vi "BusUI.vi"() -> ()   [LabVIEW 2014, in "Bus.lvclass"]
doc: "UI that will be called when the node is selected."
uses:
  Bus.lvclass
  <vilib>/NI/Configuration Framework/Node/NodeRef.ctl
  <vilib>/NI/Configuration Framework/Node/NISE_CEF_Node.lvclass
  <vilib>/NI/AMC/Message Queue.ctl
  <vilib>/NI/AMC/Message.ctl
  <vilib>/NI/Tools/Keyed Array/KeyedArray.ctl
  <vilib>/NI/Configuration Framework/Node/UserEventRef.ctl
  <vilib>/NI/Configuration Framework/Controls/EventCluster.ctl
  RIO Target/RIO Target.lvclass
  <vilib>/NI/Configuration Framework/Node/NISE_CEF_Node.lvclass/NISE_CEF_Node.ctl
  Bus.lvclass/Bus.ctl
  Bus Configuration/SPI Configuration.ctl
  Bus Configuration/Bus Configuration.lvclass/Bus Configuration.ctl
  <vilib>/NI/AMC/Create Single Message.vi
  <vilib>/NI/AMC/Update Message Routing Info.vi
  <vilib>/NI/AMC/Send Message.vi
  <vilib>/NI/AMC/AMC.lvlib
  <vilib>/NI/Configuration Framework/serializable configuration/NISE_CEF_serializable configuration.lvclass
  Bus Configuration/Bus Configuration.lvclass
  <vilib>/NI/Tools/Keyed Array/Tools_KeyedArray.lvlib
  <vilib>/NI/Configuration Framework/NISE_CEF_TreeControl.lvlib
panel:
  in  "Comments":string
  in  "SPI Engine":path
  in  "Driver Logic Unit":path
  in  "MOSI":string(combo)
  in  "MISO":string(combo)
  in  "SCLK":string(combo)
  in  "Alias":string
  in  "Replace Default SPI Engine?":bool
  in  "Replace Default DLU?":bool
  in  "user event":T1
  in  "main queue":T2
  in  "node ref":T3
  # "Settings"
  # "Alias"
  # "Comments"
  # "SPI Configuration"
  # "SCLK"
  # "SPI Engine"
  # "Driver Logic Unit"
  # "MOSI"
  # "MISO"
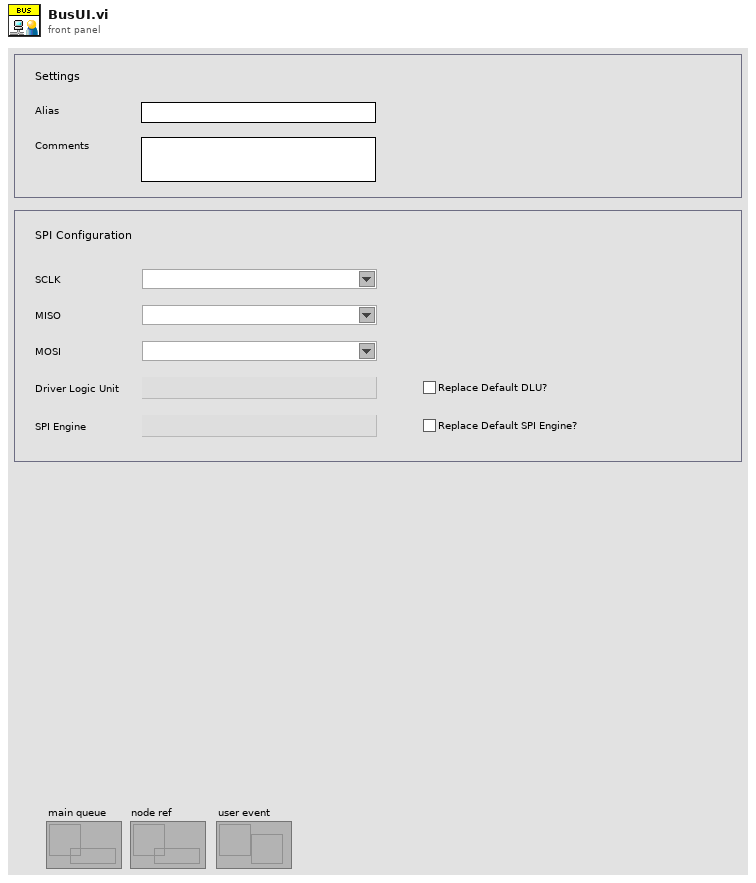
[diagram p1: front panel]
types:
  T1 = typedef "NISE_CEF_Node.lvclass/UserEventRef.ctl" = refnum<user-event>
  T2 = typedef "AMC.lvlib/Message Queue.ctl" = refnum<queue>
  T3 = typedef "NISE_CEF_Node.lvclass/NodeRef.ctl" = refnum<data-value>
  T4 = typedef "Bus.lvclass/UI Configuration.ctl" = cluster{"SPI Engine":path, "Driver Logic Unit":path, "alias":string, "SPI Configuration":T5, "Replace Default DLU?":bool, "Replace Default SPI Engine?":bool}
  T5 = typedef "Bus Configuration.lvclass/SPI Configuration.ctl" = cluster{"SCLK":string, "MOSI":string, "MISO":string}
  T6 = enum8{"Enabled", "Disabled", "Disabled and Grayed Out"}
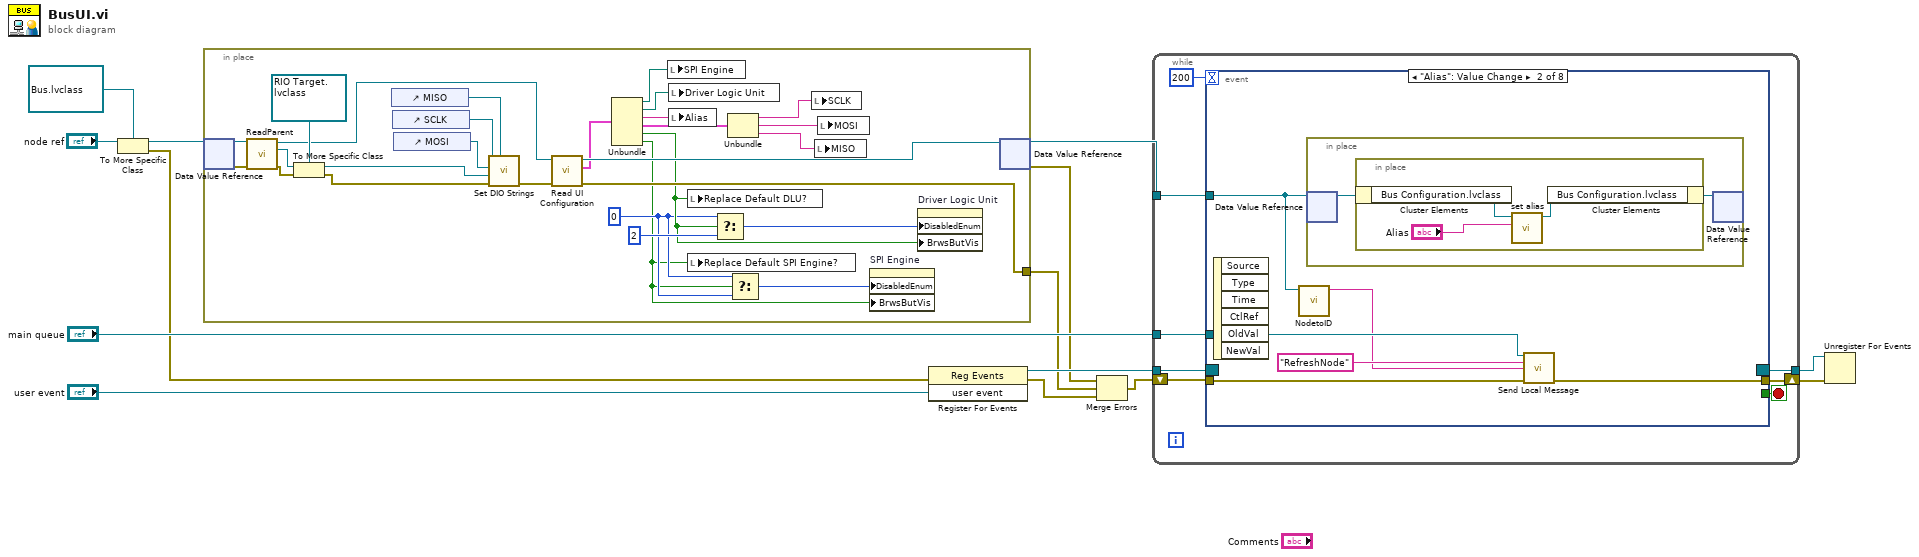
[diagram p0: block diagram]
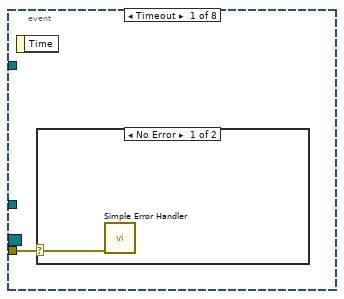
[diagram p2: hidden frame]
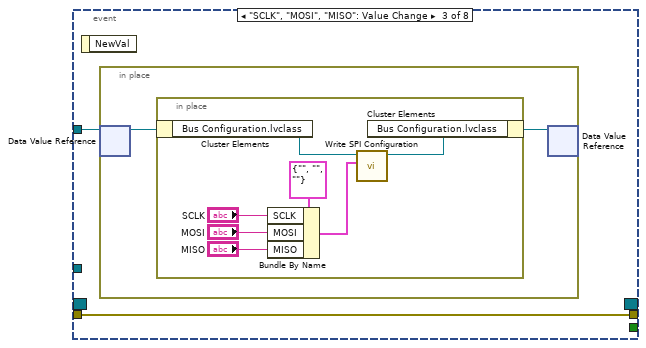
[diagram p4: hidden frame]
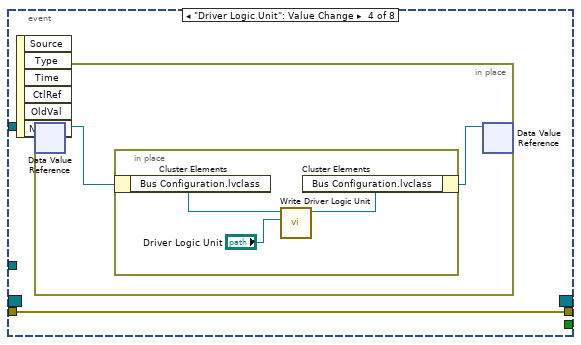
[diagram p5: hidden frame]
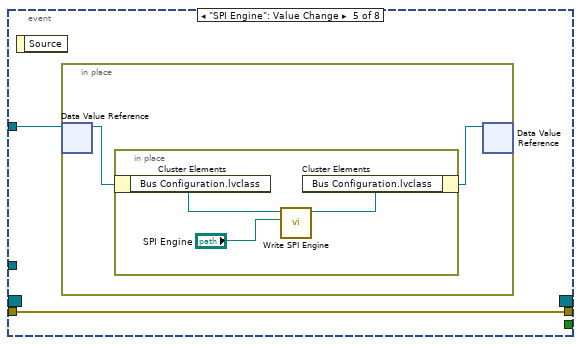
[diagram p6: hidden frame]
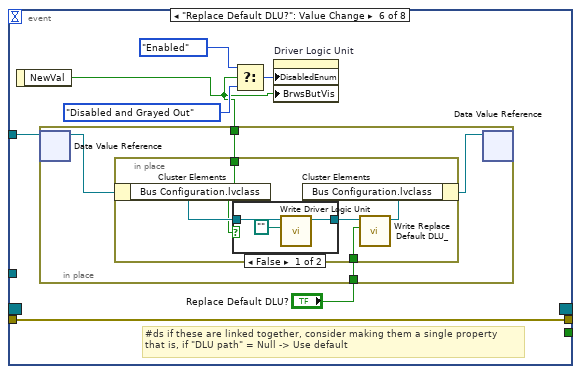
[diagram p7: hidden frame]
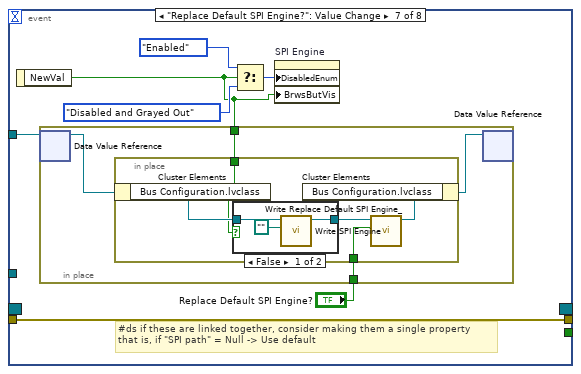
[diagram p9: hidden frame]
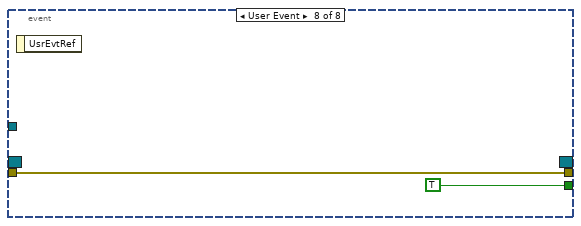
[diagram p11: hidden frame]
diagram:
  n1 = To More Specific Class(target class=refnum<data-value> refnum ("data value reference"), reference="node ref") -> (specific class reference=w5:refnum<data-value>, error out=w1:errorcluster)  [unwired: 1 in]
  n2 = in-place {
    in-place-border: [w32] -> w2
    w17 = 0
    n3 = in-place-dvr #1(w5) -> (w42:refnum<class "Bus.lvclass">, w36:errorcluster)
    n4 = call <vilib>:"ReadParent.vi"("error in"=w36, "node in"=w42) -> ("error out"=w35:errorcluster, "parent"=w41:T3, "node out"=w38:refnum<class "Bus.lvclass">)  [unwired: 7 in]
    n5 = To More Specific Class(target class=refnum<data-value> refnum ("data value reference"), reference=w41, error in=w35) -> (specific class reference=w39:refnum<data-value>, error out=w34:errorcluster)
    n6 = control-ref of="MISO"() -> (w30:refnum<vi>)
    n7 = control-ref of="SCLK"() -> (w29:refnum<vi>)
    n8 = control-ref of="MOSI"() -> (w31:refnum<vi>)
    n9 = call "Set DIO Strings.vi"("MISO"=w30, "error in (no error)"=w34, "Bus ref"=w39, "MOSI"=w31, "ComboBox in"=w29) -> ("error out"=w33:errorcluster)  [unwired: 6 in]
    n10 = call "Read UI Configuration.vi"("error in"=w33, "Bus in"=w38) -> ("error out"=w32:errorcluster, "UI Configuration"=w28:T4, "Bus out"=w37:refnum<class "Bus.lvclass">)  [unwired: 7 in]
    n11 = Unbundle(w28) -> ("SPI Engine"=w27:path, "Driver Logic Unit"=w26:path, "alias"=w25:string, "SPI Configuration"=w24:T5, "Replace Default DLU?"=w18:bool, "Replace Default SPI Engine?"=w15:bool)
    n12 = local write "SPI Engine"(w27) -> ()
    n13 = local write "Driver Logic Unit"(w26) -> ()
    n14 = local write "Alias"(w25) -> ()
    n15 = local write "Replace Default DLU?"(w18) -> ()
    n16 = local write "Replace Default SPI Engine?"(w15) -> ()
    n17 = Select(t=w17, s=w18, f=2) -> (s? t:f=w20:i32)
    n18 = Unbundle(w24) -> ("SCLK"=w23:string, "MOSI"=w22:string, "MISO"=w21:string)
    n19 = Select(t=w17, s=w15, f=w17) -> (s? t:f=w16:i32)
    n20 = local write "SCLK"(w23) -> ()
    n21 = local write "MISO"(w21) -> ()
    n22 = local write "MOSI"(w22) -> ()
    n23 = property on="SPI Engine" class="Path"("DisabledEnum"=w16, "BrwsButVis"=w15) -> ()  [unwired: 2 in, 2 out]
    n24 = property on="Driver Logic Unit" class="Path"("DisabledEnum"=w20, "BrwsButVis"=w18) -> ()  [unwired: 2 in, 2 out]
    n25 = in-place-dvr #1(w37) -> (w14:refnum<data-value>, w3:errorcluster)
  }
  n26 = register-events(error in=w1, "user event") -> (reference out=w11:refnum<event-registration>, error out=w8:errorcluster)  [unwired: 1 in]
  n27 = Merge Errors(w3, w2, w8) -> (w7:errorcluster)
  n28 = while {
    tunnel: w14 -> [w50]
    tunnel: "main queue" -> [w49]
    tunnel: w11 -> [w47]
    tunnel: [w46] -> w10
    shift-right: [w44] -> w9
    shift-left: w7 -> [w43]
    stop <- w45 stop-if-true
    n29 = event shown="[1] \"Alias\": Value Change" {
      selector: w47 -> [_ _ _ _ _ _ _ _]
      dyn-events: [_ _ _ _ _ _ _ _] -> w46
      timeout: 200 -> [_ _ _ _ _ _ _ _]
      tunnel: w50 -> [_ w56 w64 w75 w82 w94 w114 _]
      tunnel: w49 -> [_ w57 _ _ _ _ _ _]
      tunnel: [_ _ _ _ _ _ _ TRUE] -> w45
      tunnel: [_ w54 w65 w76 w83 w95 w115 w129] -> w44
      tunnel: w43 -> [w51 w53 w65 w76 w83 w95 w115 w129]
      event Timeout {
        n30 = event-data() -> ()  [unwired: 1 in, 1 out]
        n31 = case shown="No Error" w51 {
          selector: w51 -> [w52 _]
          frame No Error {
            n32 = call <vilib>:"Simple Error Handler.vi"("error in (no error)"=w52) -> ()  [unwired: 4 in, 5 out]
          }
          frame Error {
          }
        }
      }
      event "Alias": Value Change {
        n33 = event-data() -> ()  [unwired: 1 in, 6 out]
        n34 = call <vilib>:"NodetoID.vi"("node ref"=w56) -> ("ID"=w55:string)  [unwired: 9 in, 1 out]
        n35 = in-place {
          n36 = in-place-dvr #2(w56) -> (w60:refnum<class "Bus.lvclass">)  [unwired: 1 out]
          n37 = in-place {
            n38 = in-place-cluster #3(w60) -> ("Bus Configuration.lvclass"=w63:refnum<class "Bus Configuration.lvclass">)
            n39 = call <vilib>:"set alias.vi"("alias"="Alias", "configuration in"=w63) -> ("configuration out"=w62:refnum<class "Bus Configuration.lvclass">)  [unwired: 8 in, 1 out]
            n40 = in-place-cluster #3("Bus Configuration.lvclass"=w62) -> (w59:refnum<class "Bus.lvclass">)
          }
          n41 = in-place-dvr #2(w59) -> ()  [unwired: 2 out]
        }
        n42 = call <vilib>:"Send Local Message.vi"("message queue in"=w57, "message name"="RefreshNode" ("Message Name"), "message value"=w55, "error in"=w53) -> ("error out"=w54:errorcluster)  [unwired: 9 in, 2 out]
      }
      event "SCLK", "MOSI", "MISO": Value Change {
        n43 = event-data() -> ()  [unwired: 1 in, 1 out]
        n44 = in-place {
          n45 = in-place-dvr #4(w64) -> (w67:refnum<class "Bus.lvclass">)  [unwired: 1 out]
          n46 = in-place {
            n47 = in-place-cluster #5(w67) -> ("Bus Configuration.lvclass"=w74:refnum<class "Bus Configuration.lvclass">)
            n48 = Bundle By Name(cluster=T5 {"SCLK"="", "MOSI"="", "MISO"=""} ("SPI Configuration"), "SCLK"="SCLK", "MOSI"="MOSI", "MISO"="MISO") -> (w68:T5)
            n49 = call "Write SPI Configuration.vi"("SPI Configuration"=w68, "Bus Configuration in"=w74) -> ("Bus Configuration out"=w73:refnum<class "Bus Configuration.lvclass">)  [unwired: 8 in, 1 out]
            n50 = in-place-cluster #5("Bus Configuration.lvclass"=w73) -> (w66:refnum<class "Bus.lvclass">)
          }
          n51 = in-place-dvr #4(w66) -> ()  [unwired: 2 out]
        }
      }
      event "Driver Logic Unit": Value Change {
        n52 = event-data() -> ()  [unwired: 1 in, 6 out]
        n53 = in-place {
          n54 = in-place-dvr #6(w75) -> (w78:refnum<class "Bus.lvclass">)  [unwired: 1 out]
          n55 = in-place {
            n56 = in-place-cluster #7(w78) -> ("Bus Configuration.lvclass"=w81:refnum<class "Bus Configuration.lvclass">)
            n57 = call "Write Driver Logic Unit.vi"("Driver Logic Unit"="Driver Logic Unit", "Bus Configuration in"=w81) -> ("Bus Configuration out"=w80:refnum<class "Bus Configuration.lvclass">)  [unwired: 8 in, 1 out]
            n58 = in-place-cluster #7("Bus Configuration.lvclass"=w80) -> (w77:refnum<class "Bus.lvclass">)
          }
          n59 = in-place-dvr #6(w77) -> ()  [unwired: 2 out]
        }
      }
      event "SPI Engine": Value Change {
        n60 = event-data() -> ()  [unwired: 1 in, 1 out]
        n61 = in-place {
          n62 = in-place-dvr #8(w82) -> (w85:refnum<class "Bus.lvclass">)  [unwired: 1 out]
          n63 = in-place {
            n64 = in-place-cluster #9(w85) -> ("Bus Configuration.lvclass"=w88:refnum<class "Bus Configuration.lvclass">)
            n65 = call "Write SPI Engine.vi"("SPI Engine"="SPI Engine", "Bus Configuration in"=w88) -> ("Bus Configuration out"=w87:refnum<class "Bus Configuration.lvclass">)  [unwired: 8 in, 1 out]
            n66 = in-place-cluster #9("Bus Configuration.lvclass"=w87) -> (w84:refnum<class "Bus.lvclass">)
          }
          n67 = in-place-dvr #8(w84) -> ()  [unwired: 2 out]
        }
      }
      event "Replace Default DLU?": Value Change {
        # "#ds if these are linked together, consider making them a single property\nthat is, if \"DLU path\" = Null -> Use default"
        n68 = event-data() -> ("NewVal"=w90:bool)  [unwired: 1 in]
        n69 = in-place {
          in-place-border: w90 -> [w97]
          in-place-border: "Replace Default DLU?" -> [w96]
          n70 = in-place-dvr #10(w94) -> (w99:refnum<class "Bus.lvclass">)  [unwired: 1 out]
          n71 = in-place {
            in-place-border: w97 -> [w103]
            in-place-border: w96 -> [w100]
            n72 = in-place-cluster #11(w99) -> ("Bus Configuration.lvclass"=w104:refnum<class "Bus Configuration.lvclass">)
            n73 = case shown="False" w103 {
              tunnel: w104 -> [w107 w108]
              tunnel: [w106 w108] -> w102
              frame False {
                n74 = call "Write Driver Logic Unit.vi"("Driver Logic Unit"=path "", "Bus Configuration in"=w107) -> ("Bus Configuration out"=w106:refnum<class "Bus Configuration.lvclass">)  [unwired: 8 in, 1 out]
              }
              frame True {
              }
            }
            n75 = call "Write Replace Default DLU_.vi"("Replace Default DLU?"=w100, "Bus Configuration in"=w102) -> ("Bus Configuration out"=w101:refnum<class "Bus Configuration.lvclass">)  [unwired: 8 in, 1 out]
            n76 = in-place-cluster #11("Bus Configuration.lvclass"=w101) -> (w98:refnum<class "Bus.lvclass">)
          }
          n77 = in-place-dvr #10(w98) -> ()  [unwired: 2 out]
        }
        n78 = Select(t=T6."Enabled" ("Disabled"), s=w90, f=T6."Disabled and Grayed Out" ("Disabled")) -> (s? t:f=w91:T6)
        n79 = property on="Driver Logic Unit" class="Path"("DisabledEnum"=w91, "BrwsButVis"=w90) -> ()  [unwired: 2 in, 2 out]
      }
      event "Replace Default SPI Engine?": Value Change {
        # "#ds if these are linked together, consider making them a single property\nthat is, if \"SPI path\" = Null -> Use default"
        n80 = event-data() -> ("NewVal"=w110:bool)  [unwired: 1 in]
        n81 = in-place {
          in-place-border: w110 -> [w117]
          in-place-border: "Replace Default SPI Engine?" -> [w116]
          n82 = in-place-dvr #12(w114) -> (w119:refnum<class "Bus.lvclass">)  [unwired: 1 out]
          n83 = in-place {
            in-place-border: w117 -> [w123]
            in-place-border: w116 -> [w120]
            n84 = in-place-cluster #13(w119) -> ("Bus Configuration.lvclass"=w124:refnum<class "Bus Configuration.lvclass">)
            n85 = case shown="False" w123 {
              tunnel: w124 -> [w127 w128]
              tunnel: [w126 w128] -> w122
              frame False {
                n86 = call "Write SPI Engine.vi"("SPI Engine"=path "", "Bus Configuration in"=w127) -> ("Bus Configuration out"=w126:refnum<class "Bus Configuration.lvclass">)  [unwired: 8 in, 1 out]
              }
              frame True {
              }
            }
            n87 = call "Write Replace Default SPI Engine_.vi"("Replace Default SPI Engine?"=w120, "Bus Configuration in"=w122) -> ("Bus Configuration out"=w121:refnum<class "Bus Configuration.lvclass">)  [unwired: 8 in, 1 out]
            n88 = in-place-cluster #13("Bus Configuration.lvclass"=w121) -> (w118:refnum<class "Bus.lvclass">)
          }
          n89 = in-place-dvr #12(w118) -> ()  [unwired: 2 out]
        }
        n90 = Select(t=T6."Enabled" ("Disabled"), s=w110, f=T6."Disabled and Grayed Out" ("Disabled")) -> (s? t:f=w111:T6)
        n91 = property on="SPI Engine" class="Path"("DisabledEnum"=w111, "BrwsButVis"=w110) -> ()  [unwired: 2 in, 2 out]
      }
      event User Event {
        n92 = event-data() -> ()  [unwired: 1 in, 1 out]
      }
    }
  }
  n93 = Unregister For Events(event registration refnum=w10, error in=w9) -> ()  [unwired: 1 out]
